vi "AlliGator Filter Phasors in ROI(s).vi"(7 "Phasor Plot Image":T1, 8 "error in (no error)":errorcluster, 9 "All Phasor Plot ROIs":bool, 10 "Selected Phasor Plot ROI(s)":bool, 11 "Phasor Array in":csg[](array[numeric])) -> (0 "error out":errorcluster, 1 "Message":string, 3 "Phasor Array out":csg[](array[numeric]))   [LabVIEW 2021, in "AlliGator Phasor Plot.lvlib"]
doc: "Returns an array of phasor values located within the selected Phasor Plot ROI (or All ROIs)."
uses:
  AlliGator Phasor Plot.lvlib
  <vilib>/vision/Image Controls.llb/IMAQ Image.ctl
  AlliGator Variables List.ctl
  AlliGator Phasor Plot Reference Points.ctl
  91eb7ac0-7abc-46e1-b76d-bce32f8ebfb4.vi
  <userlib>/_OpenG.lib/array/array.llb/Filter 1D Array (CSG)__ogtk.vi
  AlliGator ROIs.lvlib
  <vilib>/vision/NI_Vision_Development_Module.lvlib
  AlliGator Globals, Variables & Constants.lvlib
  AlliGator Phasor Ratio.lvlib
  Strings/Strings.lvlib
  <userlib>/_OpenG.lib/array/array.llb/openg_array.lvlib
  Error/Error.lvlib
panel:
  # "see the AlliGator License on the block diagram (Ctrl+E or Window:Show Block Diagram)"
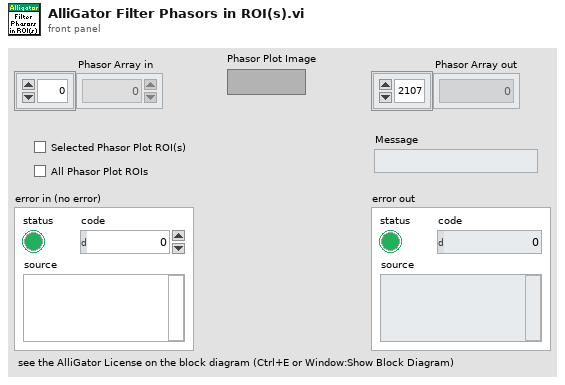
[diagram p1: front panel]
types:
  T1 = typedef "IMAQ Image.ctl" = refnum<image>
  T2 = typedef "AlliGator Phasor Ratio.lvlib/AlliGator Phasor Plot Reference Points.ctl" = cluster{"O_h":dbl, "O_v":dbl, "1_h":dbl, "1_v":dbl}
  T3 = typedef "AlliGator Globals, Variables & Constants.lvlib/AlliGator Variables List.ctl" = enum16{"---- GUI ----", "Initialization Status", "State Indicators Refnum", "Original AlliGator Menu Items", "Current Action Loop State", "Script in progress", "Playback", "Loop Playback", "Search ROI Used", "Search ROI", "Decay Graph Max Legend Size", "Intensity Graph Max Legend Size", "Decay Statistics Graph Max Legend Size", "Phasor Graph Max Legend Size", "Phasor Ratio Graph Max Legend Size", "Lifetime Graph Max Legend Size", "---- Files ----", "Export Dataset Frames as Individual Files", "Show Batch Export Help Balloons", "Frames in Dataset", "ptu File Frame Start Indices", "Current Frame in Dataset", "Current Frame Timestamp", "------ Python Plugins ------", "Python Plugins Information", "Python Session", "Valid Python Session?", "---- Source Image ----", "Dataset Loaded", "Dataset Metadata", "Dataset Channel", "Dataset Data Description", "Background Dataset Metadata", "Background Dataset Channel", "Background Dataset Data Description", "Background File Subtraction", "Background File Path", "Background File Pile-up Correction", "Background File Pixel Well Capacity", "Background File Scaling Factor", "Source Image ROIs", "Current Source Image ROI", "Source Image ROI Event Refnum", "X_Source Image Display Range", "X_Source Image Palette Information", "Source Image Palette List", "Source Image Scale", "Current Dataset Load Settings", "Source Image:ROI Overlay Color", "---- Image Profile Window ----", "Image Profile:Overlay ROI in Source Image", "Image Profile Window Event Refnum", "Image Profile:IntensityType", "Image Profile:Intensity Average Type", "Image Profile:Intensity-weighted SDV", "Image Profile:Box Profile Type", "Image Profile Window Open", "Image Profile:Plotted Fit Parameter", "X_Type of Displayed Image", "X_Time Gate Slider", "Dataset Path", "Source Image Overlay to Erase", "Is Displayed Image Accumulated", "White Light Image Modified", "Mask Image Modified", "Macrotime Gate Separation", "------ Phasor Graph -------", "Phasor Graph:Show Line", "---- Phasor Plot ---", "Phasor Plot Parameters Changed", "FLI Dataset Modified since last Phasor Plot Calculation", "Phasor Harmonics Data", "Selected Phasor Harmonics", "Phasor Harmonic Manager Event Refnum", "Phasor Plot ROIs", "Current Phasor Plot ROI", "Phasor Plot ROI Event Refnum", "Phasor Plot Image Reference Points", "Phasor Plot Computed", "Phasor Plot Palette Information", "Phasor Plot Palette List", "Phasor Ratio Palette Information", "Phasor Ratio Palette List", "Phasor Image Scale", "Phasor Plot Image Overlay to Erase", "Phasor Plot Image Elements to Update", "Current Phasor Plot Calculation Parameters", "Current Phasor Calibration Options", "Reset Cumulated Phasor Plot", "Phasor Ratio Reference 1", "Phasor Ratio Lifetime Reference 1", "Phasor Ratio Reference 1 Frequency", "Phasor Ratio Reference 2", "Phasor Ratio Lifetime Reference 2", "Phasor Ratio Reference 2 Frequency", "---- Decay Analysis ----", "Number of Selected Decays to Fit", "LS Fit Results", "LAR Fit Results", "BS Fit Results", "Last Decay Max - Min", "Best Fit Parameters", "Best Fit Parameter Names", "Actual Size X", "Actual Size Y", "Binning X", "Binning Y", "Actual # Gates", "Dataset Number", "Gates to...", "Gates Skipped", "Gates to keep", "Gate Step", "Gate Separation", "Reversed Gates", "Pile-up Correction", "Pixel Well Capacity", "Background Subtracted", "Background Subtraction Method", "Background Definition Range", "Background File (deprecated)", "Number of Dataset Accumulated", "Array of Accumulated Dataset Paths", "Do Averaged Datasets", "Destination File Path", "Process Plot Target", "Use 1/D as Phasor Frequency", "---- Decay Fit Parameter Map -----", "Decay Fit Parameter Map Palette Information", "Decay Fit Parameter Map Palette List", "Local Decay Graph Window Event Refnum", "------- Local Decay Window ---------", "Use normalized IRF for convolution", "----- Miscellaneous ----", "Skippable Dialog Windows Status"}
  T4 = typedef "Image Type" = u32
  T5 = typedef "Image.lvlib/Named ROI Description.ctl" = cluster{"ROI Descriptor":T6, "ROI Name":string, "Overlay Color":u32}
  T6 = typedef "ROI Descriptor" = cluster{"Global Rectangle":i32[], "Contours":cluster{"ID":enum32{"External", "Internal"}, "Type":u32, "Coordinates":i32[]}[]}
  T7 = cluster{"Phasor Plot x":dbl, "Phasor Plot y":dbl}
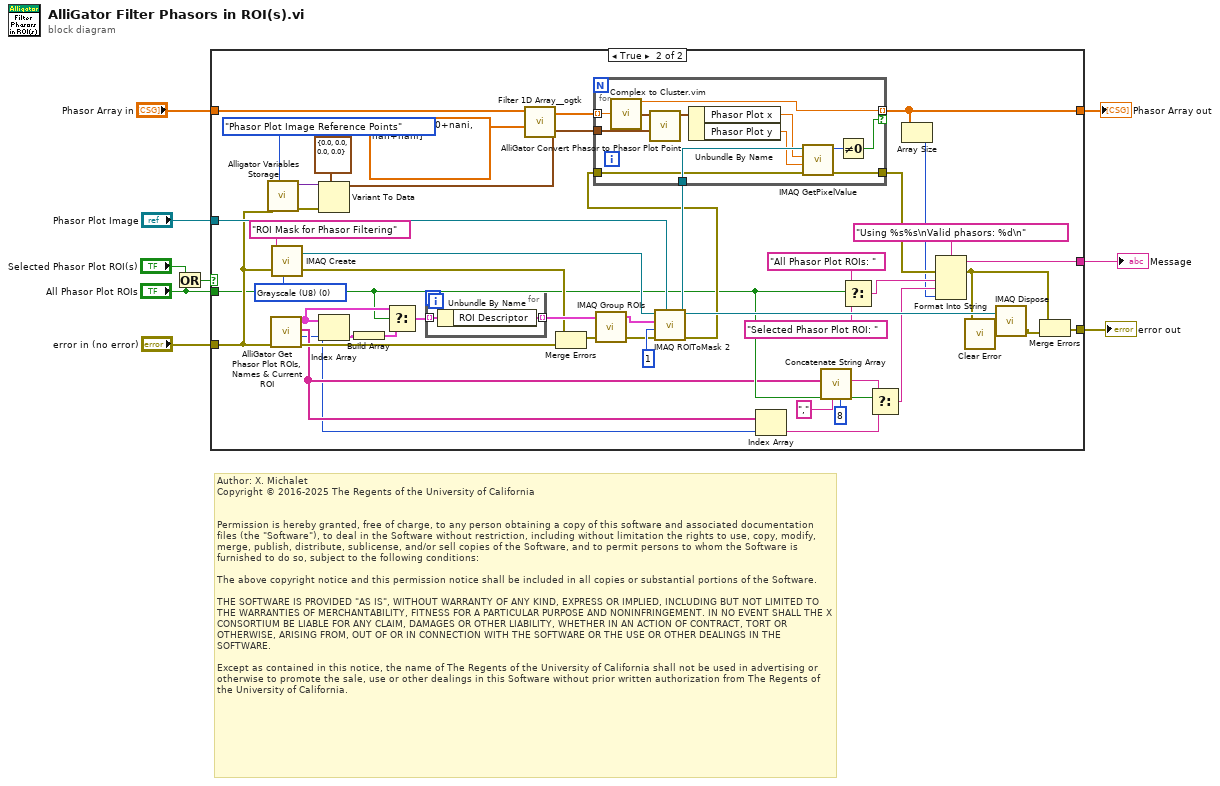
[diagram p0: block diagram]
diagram:
  # "Author: X. Michalet\nCopyright © 2016-2025 The Regents of the University of California\n \n\nPermission is hereby granted, free of charge, to any person obtaining a copy of this software and associated documentation files (the \"Software\"), to deal in the Software without restriction, including without limitation the rights to use, copy, modify, merge, publish, distribute, sublicense, and/or sell copies of the Software, and to permit persons to whom the Software is furnished to do so, subject to the following conditions:\n\nThe above copyright notice and this permission notice shall be included in all copies or substantial portions of the Software.\n\nTHE SOFTWARE IS PROVIDED \"AS IS\", WITHOUT WARRANTY OF ANY KIND, EXPRESS OR IMPLIED, INCLUDING BUT NOT LIMITED TO THE WARRANTIES OF MERCHANTABILITY, FITNESS FOR A PARTICULAR PURPOSE AND NONINFRINGEMENT. IN NO EVENT SHALL THE X CONSORTIUM BE LIABLE FOR ANY CLAIM, DAMAGES OR OTHER LIABILITY, WHETHER IN AN ACTION OF CONTRACT, TORT OR OTHERWISE, ARISING FROM, OUT OF OR IN CONNECTION WITH THE SOFTWARE OR THE USE OR OTHER DEALINGS IN THE SOFTWARE.\n\nExcept as contained in this notice, the name of The Regents of the University of California shall not be used in advertising or otherwise to promote the sale, use or other dealings in this Software without prior written authorization from The Regents of the University of California."
  n1 = Or(x="Selected Phasor Plot ROI(s)", y="All Phasor Plot ROIs") -> (x .or. y?=w6:bool)
  n2 = case shown="True" w6 {
    tunnel: "error in (no error)" -> [w10 w38]
    tunnel: "All Phasor Plot ROIs" -> [_ w22]
    tunnel: "Phasor Array in" -> [w11 w37]
    tunnel: [w11 w17] -> w4
    tunnel: [w10 w13] -> w3
    tunnel: "Phasor Plot Image" -> [_ w44]
    tunnel: [_ w31] -> w1
    frame False {
    }
    frame True {
      w56 = T4 0 items=["Grayscale (U8)", "Grayscale (I16)", "Grayscale (SGL)", "Complex (CSG)", "RGB (U32)", "HSL (U32)", "RGB (U64)", "Grayscale (U16)"] ("Image Type")
      n3 = call "Alligator Variables Storage.vi"("AlliGator Variable"=AlliGator_Variables_List."Phasor Plot Image Reference Points" ("Alligator Variable"), "Error In"=w38) -> ("Error Out"=w40:errorcluster, "Data out"=w41:variant)  [unwired: 7 in, 1 out]
      n4 = call "AlliGator Get Phasor Plot ROIs, Names & Current ROI.vi"("Error In"=w38) -> ("Error Out"=w48:errorcluster, "Current ROI"=w20:i32, "ROI Names"=w21:string[], "Stored ROIs"=w51:T5[])  [unwired: 7 in]
      n5 = call "IMAQ Create"("Image Name"="ROI Mask for Phasor Filtering", "Image Type"=w56, "error in (no error)"=w38) -> ("New Image"=w45:T1, "error out"=w46:errorcluster)  [unwired: 2 in]
      n6 = Variant To Data(error in=w40, type=T2 {"O_h"=0.0, "O_v"=0.0, "1_h"=0.0, "1_v"=0.0} ("Phasor Plot Reference Points"), Variant=w41) -> (data=w35:T2)  [unwired: 1 out]
      n7 = Index Array(array=w51, index=w20) -> (element=w55:T5)
      n8 = Build Array(w55) -> (w54:T5[])
      n9 = Select(t=w51, s=w22, f=w54) -> (s? t:f=w50:T5[])
      n10 = for {
        tunnel: w50 -> [w70] mode=indexing
        tunnel: [w69] -> w49 mode=indexing
        n11 = Unbundle By Name(w70) -> ("ROI Descriptor"=w69:T6)
      }
      n12 = call-poly <userlib>:"Filter 1D Array__ogtk.vi"("items to filter"=csg[] [nan+0.0i, 0.0+nani, nan+nani] ("Element(s) to Remove"), "array"=w37) -> ("filtered array"=w34:csg[])  [unwired: 4 in, 1 out]
      n13 = Merge Errors(w46, w48) -> (w47:errorcluster)
      n14 = call "IMAQ Group ROIs"("error in (no error)"=w47, "ROI Descriptors"=w49) -> ("error out"=w52:errorcluster, "ROI Descriptor out"=w43:T6)  [unwired: 2 in]
      n15 = call "IMAQ ROIToMask 2"("Image Model"=w44, "error in (no error)"=w52, "Filling Value (255)"=1, "ROI Descriptor"=w43, "Image"=w45) -> ("error out"=w32:errorcluster, "Image Out"=w33:T1)  [unwired: 4 in, 1 out]
      n16 = for {
        tunnel: w35 -> [w68]
        tunnel: w34 -> [w66] mode=indexing
        tunnel: [w66] -> w17 mode=indexing if=w59
        tunnel: w33 -> [w65]
        tunnel: w32 -> [w61]
        tunnel: [w58] -> w30
        n17 = call "Complex to Cluster.vim"("x + iy"=w66) -> ("Complex Coordinates"=w67:cluster{sgl, sgl})  [unwired: 8 in]
        n18 = call "AlliGator Convert Phasor to Phasor Plot Point.vi"("Phasor Plot Reference Points"=w68, "Phasor"=w67) -> ("Phasor Plot Point"=w64:T7)  [unwired: 9 in]
        n19 = Unbundle By Name(w64) -> ("Phasor Plot x"=w63:dbl, "Phasor Plot y"=w62:dbl)
        n20 = call "IMAQ GetPixelValue"("Image"=w65, "X Coordinate"=w63, "Y Coordinate"=w62, "error in (no error)"=w61) -> ("Pixel Value (U8)"=w60:u8, "error out"=w58:errorcluster)  [unwired: 2 in, 3 out]
        n21 = Not Equal To 0?(x=w60) -> (x != 0?=w59:bool)
      }
      n22 = Index Array(array=w21, index=w20) -> (element=w19:string)
      n23 = call "Concatenate String Array.vi"("Max Number of Elements (None: -1)"=8, "Separator (TAB)"=",", "String Array"=w21) -> ("Formatted String"=w23:string)  [unwired: 8 in]
      n24 = Select(t="All Phasor Plot ROIs: " ("format string"), s=w22, f="Selected Phasor Plot ROI: " ("format string")) -> (s? t:f=w26:string)
      n25 = Select(t=w23, s=w22, f=w19) -> (s? t:f=w18:string)
      n26 = Array Size(array=w17) -> (size(s)=w16:i32)
      n27 = Format Into String(format string="Using %s%s\nValid phasors: %d\n", error in=w30, w26, w18, w16) -> (resulting string=w31:string, error out=w14:errorcluster)  [unwired: 1 in]
      n28 = call "Clear Error.vi"("Error In"=w14) -> ("no Error Out"=w12:errorcluster)  [unwired: 8 in]
      n29 = call "IMAQ Dispose"("Image"=w33, "error in (no error)"=w12) -> ("error out"=w15:errorcluster)  [unwired: 4 in]
      n30 = Merge Errors(w14, w15) -> (w13:errorcluster)
    }
  }
  "Phasor Array out" <- w4
  "error out" <- w3
  "Message" <- w1
